vi "ProjectLabView.vi"() -> ()   [LabVIEW 2025]
uses:
  <vilib>/Instr/_visa.llb/VISA Configure Serial Port (Instr).vi
panel:
  out "MIXED COLORS":u32(colorbox)
  out "concatenated string":string
  in  "BLUE PWM":u8(slide) scale=0.0..255.0
  in  "GREEN PWM":u8(slide) scale=0.0..255.0
  in  "RED PWM":u8(slide) scale=0.0..255.0
  in  "BLUE":bool
  in  "GREEN":bool
  in  "RED":bool
  out "Pico Response":string
  out "return count":u32
  in  "stop":bool
  in  "VISA resource name":refnum<visa-resource-name>
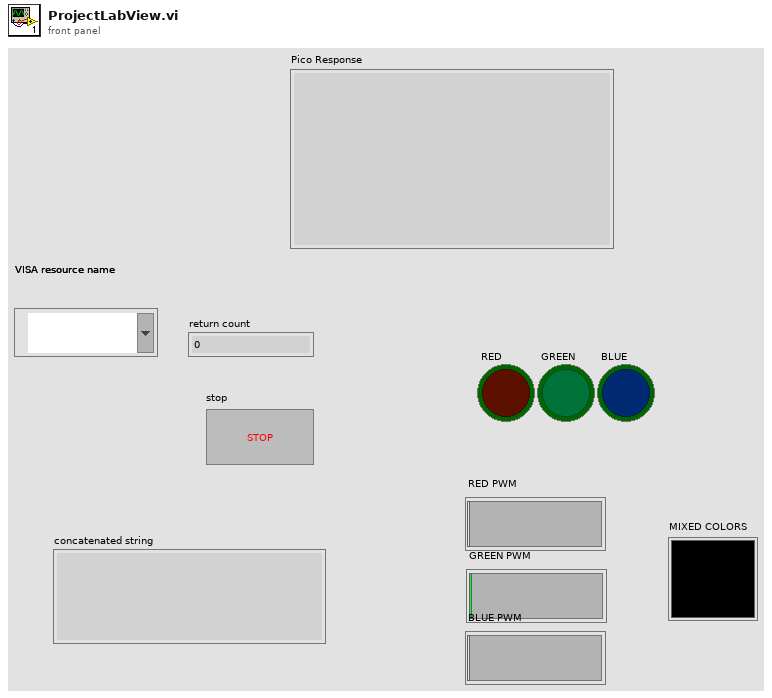
[diagram p1: front panel]
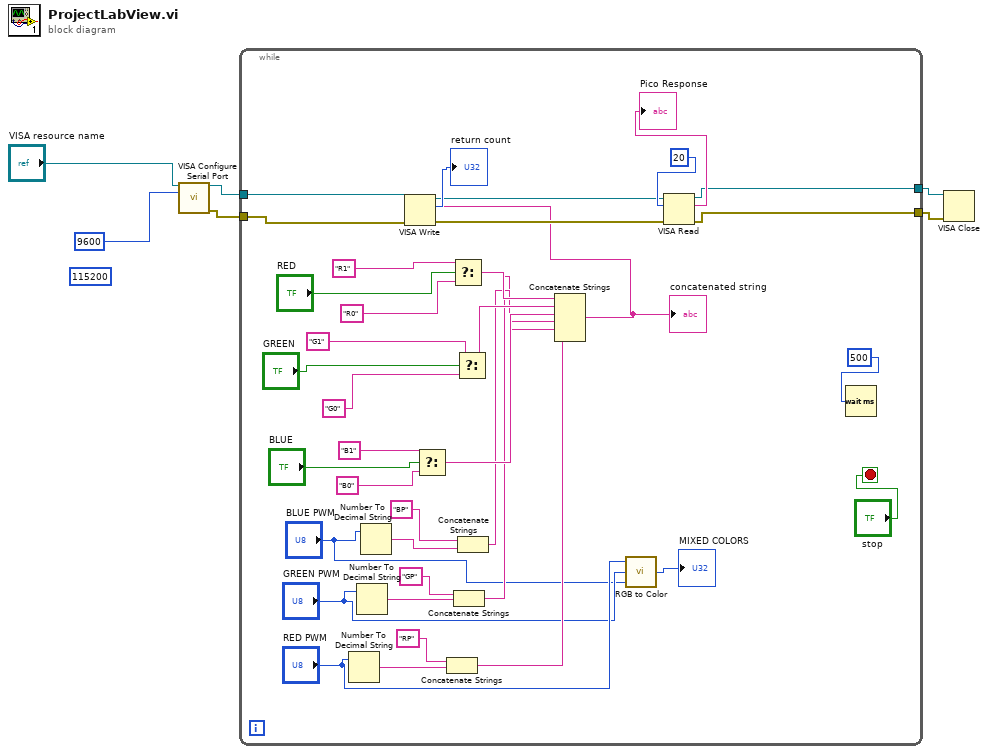
[diagram p0: block diagram]
diagram:
  (unwired) u32 115200 ("baud rate (9600)")
  n1 = call-poly "VISA Configure Serial Port"("VISA resource name"="VISA resource name", "baud rate (9600)"=u32 9600) -> ("VISA resource name out"=w6:refnum<visa-resource-name>, "error out"=w5:errorcluster)  [unwired: 12 in]
  n2 = while {
    tunnel: w6 -> [w41]
    tunnel: w5 -> [w40]
    tunnel: [w37] -> w4
    tunnel: [w36] -> w3
    stop <- "stop" stop-if-true
    n3 = Number To Decimal String(number="RED PWM") -> (decimal integer string=w16:string)  [unwired: 1 in]
    n4 = Number To Decimal String(number="GREEN PWM") -> (decimal integer string=w17:string)  [unwired: 1 in]
    n5 = Number To Decimal String(number="BLUE PWM") -> (decimal integer string=w19:string)  [unwired: 1 in]
    n6 = Select(t="B1", s="BLUE", f="B0") -> (s? t:f=w23:string)
    n7 = Concatenate Strings("RP", w16) -> (w13:string)
    n8 = Select(t="R1", s="RED", f="R0") -> (s? t:f=w29:string)
    n9 = Concatenate Strings("GP", w17) -> (w14:string)
    n10 = Select(t="G1", s="GREEN", f="G0") -> (s? t:f=w28:string)
    n11 = Concatenate Strings("BP", w19) -> (w15:string)
    n12 = Concatenate Strings(w29, w28, w23, w15, w14, w13) -> (w30:string)
    "concatenated string" <- w30
    n13 = VISA Write(VISA resource name=w41, write buffer=w30, error in (no error)=w40) -> (VISA resource name out=w34:refnum<visa-resource-name>, return count=→"return count":u32, error out=w33:errorcluster)
    n14 = call <vilib>:"RGB to Color.vi"("B"="BLUE PWM", "G"="GREEN PWM", "R"="RED PWM") -> ("Color"=→"MIXED COLORS":u32)
    n15 = VISA Read(VISA resource name=w34, byte count=u32 20, error in (no error)=w33) -> (VISA resource name out=w36:refnum<visa-resource-name>, read buffer=→"Pico Response":string, error out=w37:errorcluster)  [unwired: 1 out]
    n16 = Wait (ms)(milliseconds to wait=u32 500) -> ()  [unwired: 1 out]
  }
  n17 = VISA Close(VISA resource name=w3, error in (no error)=w4) -> ()  [unwired: 1 out]
